vi "Wait-for-message.vi"(8 "error in (no error)":errorcluster, 11 "Client in":T1) -> (0 "error out":errorcluster, 1 "New message?":bool, 2 "Message":refnum<class "Message.lvclass">, 3 "Client out":T1)   [LabVIEW 2013, in "CameraVision.lvlib" / "CV-Client.lvclass"]
doc: "Monitors the incomming communication channel (client channel) for new messages.\nThe monitoring will timeout based on the 'Heartbeat interval' parameter in the client settings. The timeout time is 80% of the heartbeat interval value, to allow the client to send a heartbeat message and have it processed by the server. The heartbeat is separate functionality, acessed through the 'Send-heartbeat' function."
uses:
  CV-Client.lvclass
  Object-reference.ctl
  SA-SLMAPI/Sources/Message.lvclass
  CV-Client.lvclass/CV-Client.ctl
  Read Client channel.vi
  Read Heartbeat interval.vi
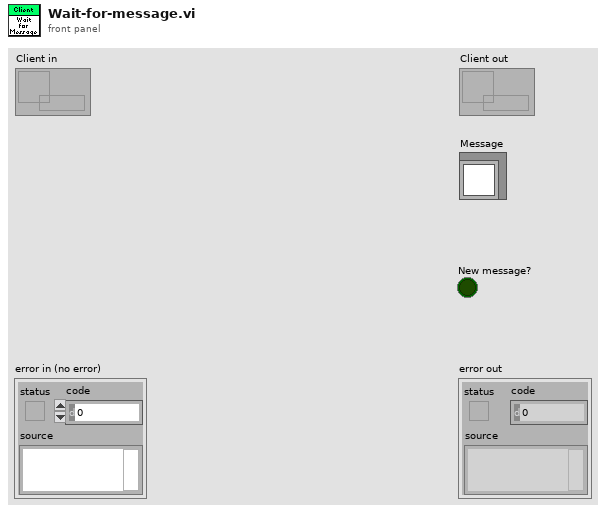
[diagram p1: front panel]
types:
  T1 = typedef "CameraVision.lvlib/CV-Client.lvclass/Object-reference.ctl" = refnum<data-value>
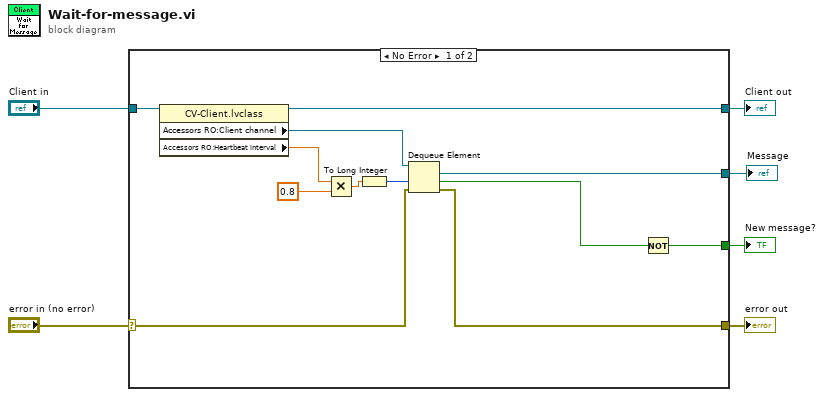
[diagram p0: block diagram]
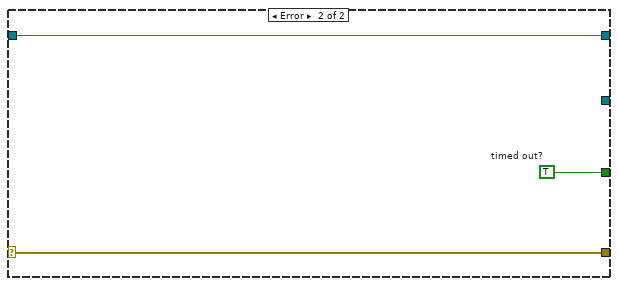
[diagram p2: hidden frame]
diagram:
  n1 = case shown="No Error" "error in (no error)" {
    selector: "error in (no error)" -> [w16 w21]
    tunnel: [w7 w21] -> w5
    tunnel: [w17 w20] -> w3
    tunnel: "Client in" -> [w18 w20]
    tunnel: [w12 w19] -> w2
    tunnel: [w13 _] -> w1
    frame No Error {
      n2 = property class="CV-Client.lvclass"(reference=w18) -> (reference out=w17:T1, "Accessors RO:Client channel"=w15:refnum<queue>, "Accessors RO:Heartbeat interval"=w11:dbl)  [unwired: 1 in, 1 out]
      n3 = Multiply(x=w11, y=0.8) -> (x*y=w10:dbl)
      n4 = To Long Integer(number=w10) -> (32bit integer=w8:i32)
      n5 = Dequeue Element(queue=w15, timeout in ms (-1)=w8, error in (no error)=w16) -> (element=w13:refnum<class "Message.lvclass">, timed out?=w14:bool, error out=w7:errorcluster)  [unwired: 1 out]
      n6 = Not(x=w14) -> (.not. x?=w12:bool)
    }
    frame Error {
      w19 = TRUE  # timed out?
    }
  }
  "error out" <- w5
  "Client out" <- w3
  "New message?" <- w2
  "Message" <- w1
